vi "Configure Output Impedance.vi"(8 "error in (no error)":errorcluster, 9 "User-Defined Impedance (50 Ohms)":dbl=50.0 min=1.0 max=10000.0 format="%.2f", 10 "Impedance (0: 50 Ohms)":u16(ring) items=["50 Ohms", "High Impedance", "User Defined"], 11 "VISA resource name":refnum<visa-resource-name>) -> (0 "error out":errorcluster, 3 "VISA resource name out":refnum<visa-resource-name>)   [LabVIEW 2018, in "AWG.lvlib" / "Agilent 33XXX Series.lvlib"]
doc: "Configures the output impedance for the function generator."
uses:
  Agilent 33XXX Series.lvlib
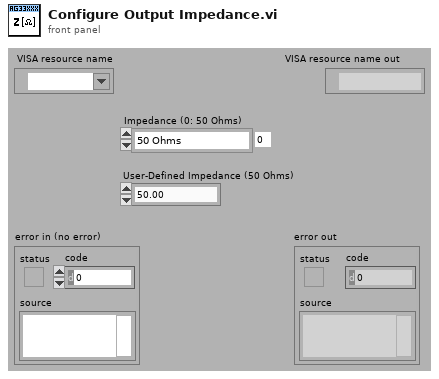
[diagram p1: front panel]
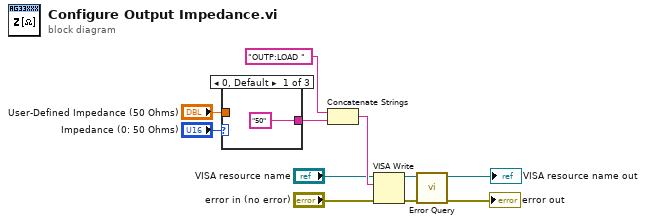
[diagram p0: block diagram]
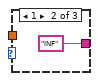
[diagram p2: hidden frame]
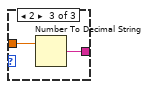
[diagram p3: hidden frame]
diagram:
  n1 = case shown="0, Default" "Impedance (0: 50 Ohms)" {
    tunnel: ["50" "INF" w15] -> w5
    tunnel: "User-Defined Impedance (50 Ohms)" -> [_ _ w14]
    frame 0, Default {
    }
    frame 1 {
    }
    frame 2 {
      n2 = Number To Decimal String(number=w14) -> (decimal integer string=w15:string)  [unwired: 1 in]
    }
  }
  n3 = Concatenate Strings("OUTP:LOAD ", w5) -> (w6:string)
  n4 = VISA Write(VISA resource name="VISA resource name", write buffer=w6, error in (no error)="error in (no error)") -> (VISA resource name out=w11:refnum<visa-resource-name>, error out=w10:errorcluster)  [unwired: 1 out]
  n5 = call "Error Query.vi"("error in (no error)"=w10, "VISA resource name"=w11) -> ("error out"=→"error out":errorcluster, "VISA resource name out"=→"VISA resource name out":refnum<visa-resource-name>)  [unwired: 6 in, 2 out]
